vi "Fetch tag.vi"() -> ()   [LabVIEW 2020]
panel:
  out "error out":errorcluster
  out "Value":string
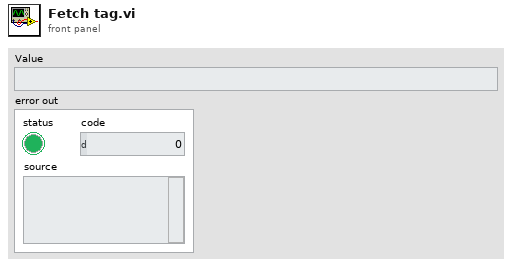
[diagram p1: front panel]
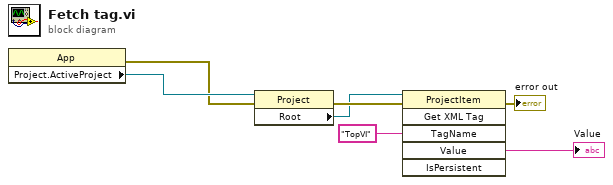
[diagram p0: block diagram]
diagram:
  n1 = property class="App"() -> (error out=w3:errorcluster, "Project.ActiveProject"=w4:refnum<vi>)  [unwired: 2 in, 1 out]
  n2 = property class="Project"(reference=w4, error in=w3) -> (error out=w7:errorcluster, "Root"=w6:refnum<vi>)  [unwired: 1 out]
  n3 = invoke class="ProjectItem" method="Get XML Tag"(reference=w6, error in=w7, "TagName"="TopVI" ("Tag Name")) -> (error out=→"error out":errorcluster, "Value"=→"Value":string)  [unwired: 3 in, 4 out]
